vi "Write FillWeight.vi"(8 "error in (no error)":errorcluster, 10 "FillWeight":sgl=1.0 min=1 max=100, 11 "GridColumn in":refnum<class "GridColumn.lvclass">) -> (0 "error out":errorcluster, 3 "GridColumn out":refnum<class "GridColumn.lvclass">)   [LabVIEW 2014, in "DataGrid.lvlib" / "GridColumn.lvclass"]
doc: "The fill weight is needed ONLY when using a FILL as autosize for columns. All fills that are used should total up to 100% so that the spacing is properly spread out to all fill columns"
uses:
  GridColumn.lvclass
  GridColumn.lvclass/GridColumn.ctl
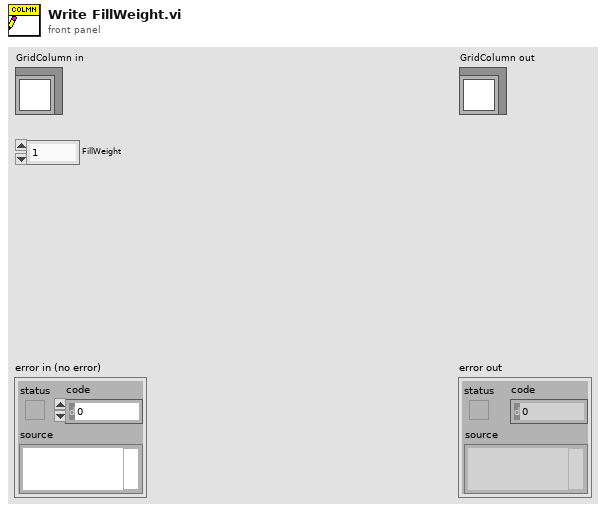
[diagram p1: front panel]
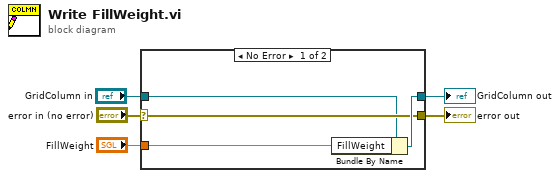
[diagram p0: block diagram]
diagram:
  n1 = case shown="No Error" "error in (no error)" {
    selector: "error in (no error)" -> [w7 w10]
    tunnel: [w7 w10] -> w4
    tunnel: [w9 w11] -> w2
    tunnel: "GridColumn in" -> [w6 w11]
    tunnel: "FillWeight" -> [w8 _]
    frame No Error {
      n2 = Bundle By Name(cluster=w6, "FillWeight"=w8) -> (w9:refnum<class "GridColumn.lvclass">)
    }
    frame Error {
    }
  }
  "error out" <- w4
  "GridColumn out" <- w2
